vi "Data Save Selection.vi"(0 "Spectral Raw Data in":refnum<class "Data.lvclass">, 1 "RR Intensity Data in":refnum<class "Data.lvclass">, 2 "RR Complex Data in":refnum<class "Complex Data.lvclass">, 3 "error in (no error)":errorcluster, 4 "Data Save Type":u16(ring) items=["RR Complex", "RR Intensity", "RAW"]) -> (5 "Data out":csg[][](array[numeric]), 6 "error out":errorcluster)   [LabVIEW 2018]
uses:
  SpectralRadar/LabVIEW/2012/user.lib/SpectralRadar.llb/Complex Data.lvclass
  SpectralRadar/LabVIEW/2012/user.lib/SpectralRadar.llb/Data.lvclass
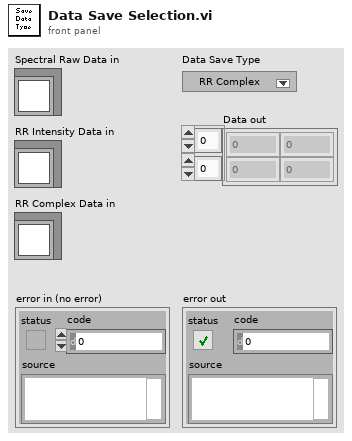
[diagram p1: front panel]
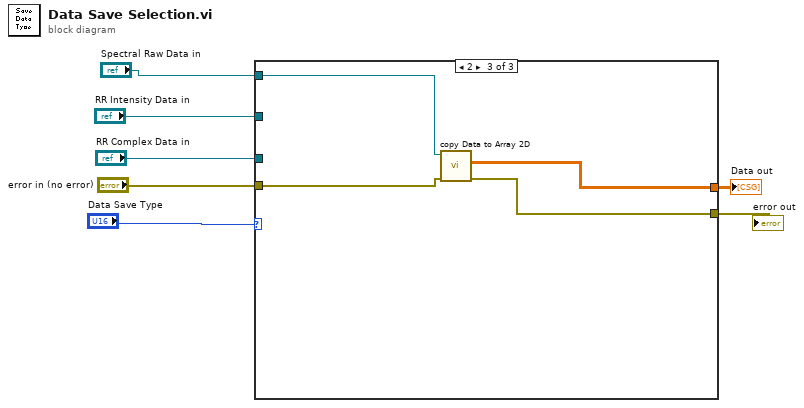
[diagram p0: block diagram]
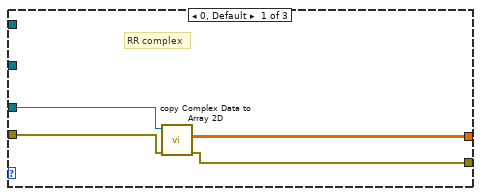
[diagram p2: hidden frame]
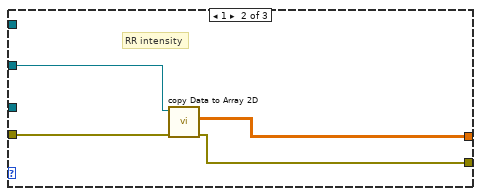
[diagram p3: hidden frame]
diagram:
  n1 = case shown="2" "Data Save Type" {
    tunnel: "RR Complex Data in" -> [w11 _ _]
    tunnel: [w10 w13 w17] -> w3
    tunnel: "error in (no error)" -> [w9 w15 w18]
    tunnel: "RR Intensity Data in" -> [_ w14 _]
    tunnel: [w8 w12 w16] -> w2
    tunnel: "Spectral Raw Data in" -> [_ _ w19]
    frame 0, Default {
      # "RR complex"
      n2 = call "copy Complex Data to Array 2D.vi"("error in (no error)"=w9, "Complex Data"=w11) -> ("error out"=w8:errorcluster, "Data Content"=w10:csg[][])  [unwired: 3 in, 1 out]
    }
    frame 1 {
      # "RR intensity"
      n3 = call "copy Data to Array 2D.vi"("error in (no error)"=w15, "Data in"=w14) -> ("error out"=w12:errorcluster, "Data Content"=w13:sgl[][])  [unwired: 3 in, 1 out]
    }
    frame 2 {
      n4 = call "copy Data to Array 2D.vi"("error in (no error)"=w18, "Data in"=w19) -> ("error out"=w16:errorcluster, "Data Content"=w17:sgl[][])  [unwired: 3 in, 1 out]
    }
  }
  "Data out" <- w3
  "error out" <- w2
